vi "ts_tree_set_section_status.vi"(8 "error in (no error)":errorcluster, 9 "ts.status":bool, 10 "ts.data":T1, 11 "Tree.in":refnum<vi>) -> (0 "error out":errorcluster, 3 "Tree.out":refnum<vi>)   [LabVIEW 2015]
doc: "sets the status symbol (pass/fail glyph) for a given active tag"
uses:
  ts-data.ctl
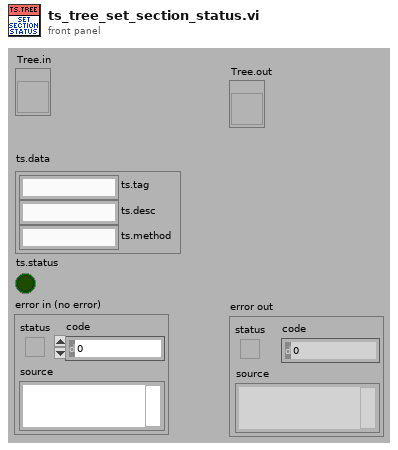
[diagram p1: front panel]
types:
  T1 = typedef "ts-data.ctl" = cluster{"ts.tag":string, "ts.desc":string, "ts.method":string}
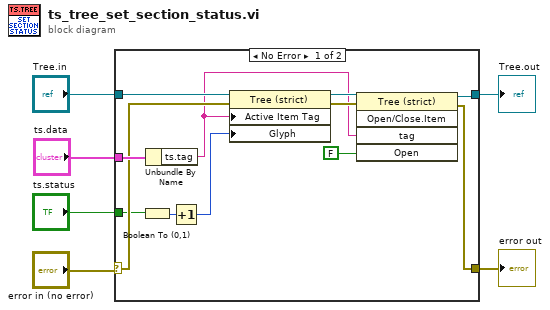
[diagram p0: block diagram]
diagram:
  n1 = case shown="No Error" "error in (no error)" {
    selector: "error in (no error)" -> [w16 w19]
    tunnel: "Tree.in" -> [w18 w20]
    tunnel: [w9 w20] -> w4
    tunnel: [w8 w19] -> w3
    tunnel: "ts.data" -> [w17 _]
    tunnel: "ts.status" -> [w15 _]
    frame No Error {
      n2 = Boolean To (0,1)(Boolean=w15) -> (0, 1=w14:i16)
      n3 = Unbundle By Name(w17) -> ("ts.tag"=w10:string)
      n4 = Increment(x=w14) -> (x+1=w13:i16)
      n5 = property class="Tree (strict)"(reference=w18, error in=w16, "Active Item Tag"=w10, "Glyph"=w13) -> (reference out=w12:refnum<vi>, error out=w11:errorcluster)
      n6 = invoke class="Tree (strict)" method="Open/Close.Item"(reference=w12, error in=w11, "tag"=w10, "Open"=FALSE ("Open?")) -> (reference out=w9:refnum<vi>, error out=w8:errorcluster)  [unwired: 1 in, 3 out]
    }
    frame Error {
    }
  }
  "Tree.out" <- w4
  "error out" <- w3
